vi "test_numpy.vi"() -> ()   [LabVIEW 2019]
uses:
  <vilib>/Analysis/Matrix/Datatypes/RealMatrix.ctl
  Ctrl/cmd_common.ctl
  <vilib>/Analysis/Matrix/Numeric/Add/Add (Elementwise) - RM,R.vi
  <vilib>/Analysis/Matrix/NI_Matrix.lvlib
  <vilib>/ptbypt/NI_PtbyPt.lvlib
panel:
  in  "sample length":i32=100
  out "Waveform Chart":cluster{dbl, dbl, "mean":dbl}(graph)
  in  "dt":u32
  in  "stop":bool
  in  "amplitude":dbl=1.0 format="%0.3f"
  out "first subarray":i32[](array[numeric])
  in  "Numeric":i32
  out "Real Matrix Element":dbl
  out "전치 행렬":T1
  out "열의 개수":i32
  out "크기 조정된 행렬":T1
  out "pw":T1=[[0.01, 0.01, 0.01, 0.01, 0.01, 0.01, 0.01, 0.01, 0.01, 0.01, 0.01, 0.01, 0.01, 0.01, 0.01, 0.01, 0.01, 0.01, 0.01, 0.01, 0.01, 0.01, 0.01, 0.01, 0.01, 0.01, 0.01, 0.01, 0.01, 0.01, 0.01, 0.01, 0.01, 0.01, 0.01, 0.01, 0.01, 0.01, 0.01, 0.01, 0.01, 0.01, 0.01, 0.01, 0.01, 0.01, 0.01, 0.01, 0.01, 0.01, 0.01, 0.01, 0.01, 0.01, 0.01, 0.01, 0.01, 0.01, 0.01, 0.01, 0.01, 0.01, 0.01, 0.01, 0.01, 0.01, 0.01, 0.01, 0.01, 0.01, 0.01, 0.01, 0.01, 0.01, 0.01, 0.01, 0.01, 0.01, 0.01, 0.01, 0.01, 0.01, 0.01, 0.01, 0.01, 0.01, 0.01, 0.01, 0.01, 0.01, 0.01, 0.01, 0.01, 0.01, 0.01, 0.01, 0.01, 0.01, 0.01, 0.01]]
  out "px":T1
  in  "NP":u32=100
  out "y 제곱근(x)":dbl
  out "x^y":dbl
  in  "**":dbl
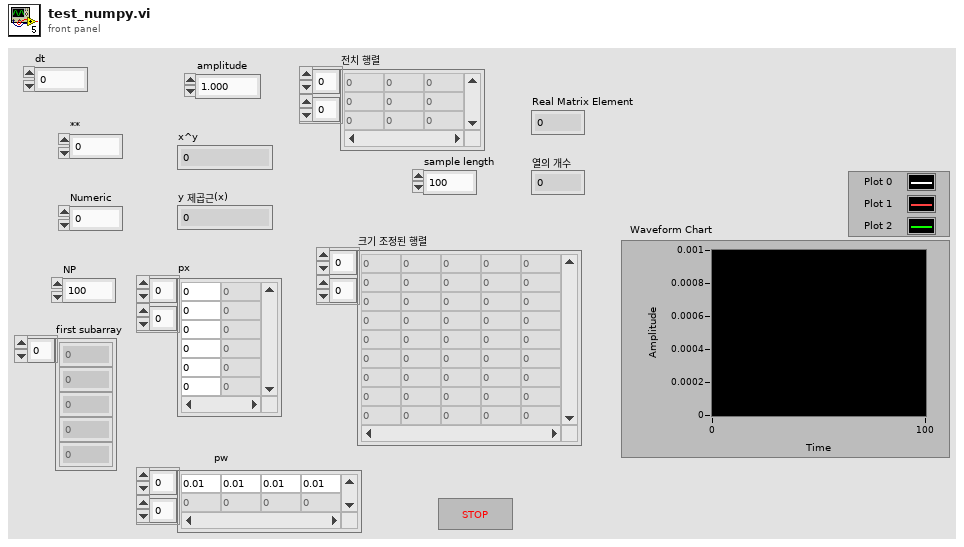
[diagram p1: front panel]
types:
  T1 = typedef "NI_Matrix.lvlib/RealMatrix.ctl" = dbl[][]
  T2 = typedef "cmd_common.ctl" = enum16{"read", "write"}
  T3 = cluster{"px":T1, "pw":T1, "x_dr":T1, "x_est":T1, "x_true":T1, "u":T1, "z":T1}
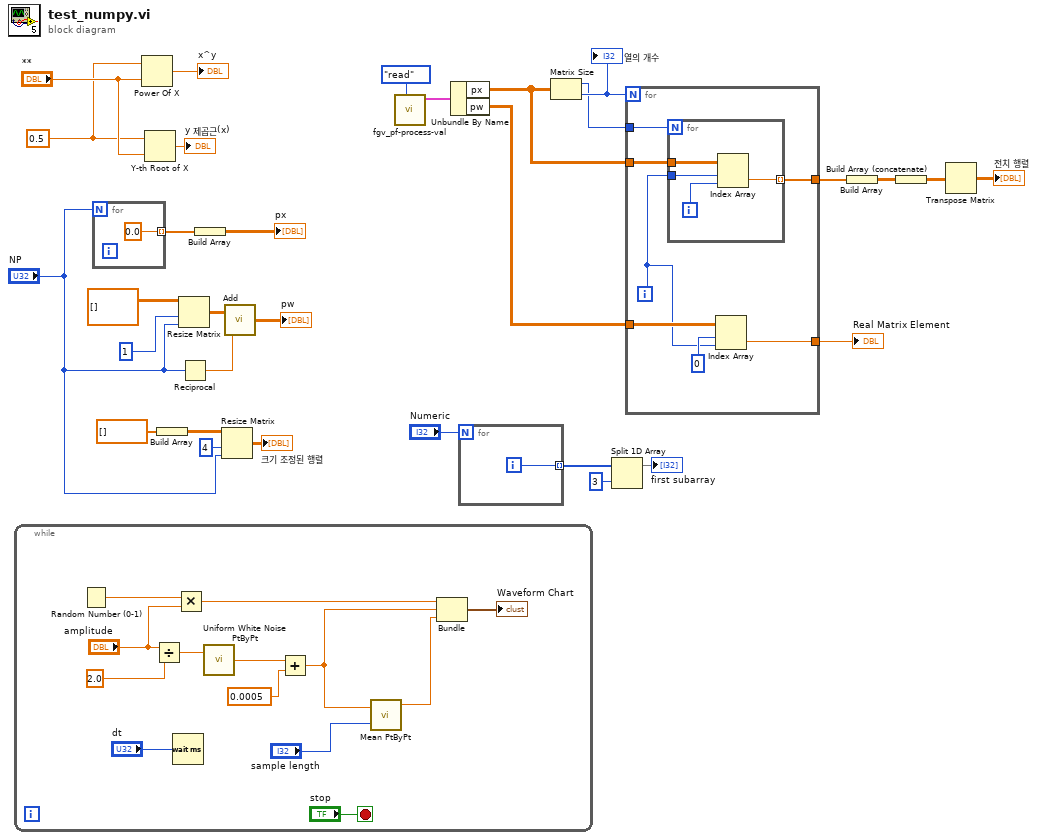
[diagram p0: block diagram]
diagram:
  w28 = 0.5 ("x")
  n1 = while {
    stop <- "stop" stop-if-true
    n2 = Random Number (0-1)() -> (number: 0 to 1=w44:dbl)
    n3 = Divide(x="amplitude", y=2.0) -> (x/y=w36:dbl)
    n4 = Wait (ms)(milliseconds to wait="dt") -> ()  [unwired: 1 out]
    n5 = Multiply(x=w44, y="amplitude") -> (x*y=w43:dbl)
    n6 = call <vilib>:"Uniform White Noise PtByPt.vi"("amplitude"=w36) -> ("uniform white noise"=w35:dbl)  [unwired: 2 in]
    n7 = Add(x=w35, y=0.0005) -> (x+y=w34:dbl)
    n8 = call <vilib>:"Mean PtByPt.vi"("x"=w34, "sample length"="sample length") -> ("mean"=w33:dbl)  [unwired: 2 in, 1 out]
    n9 = Bundle(w43, w34, "mean"=w33) -> (→"Waveform Chart":cluster{dbl, dbl, "mean":dbl})  [unwired: 1 in]
  }
  n10 = for {
    N: "NP" -> [_]
    tunnel: [0.0] -> w24 mode=indexing
  }
  n11 = Power Of X(1:"**", 2:w28) -> (0:→"x^y":dbl)
  n12 = Y-th Root of X(1:"**", 2:w28) -> (0:→"y 제곱근(x)":dbl)
  n13 = Build Array(dbl[] [] ("원소")) -> (w19:T1)
  n14 = Resize Matrix(1:"NP", 2:1 ("행의 개수"), 4:T1 [] ("행렬")) -> (0:w27:T1)
  n15 = Reciprocal(x="NP") -> (1/x=w26:dbl)
  n16 = Build Array(w24) -> (→"px":T1)
  n17 = Resize Matrix(1:"NP", 2:4 ("행의 개수"), 4:w19) -> (0:→"크기 조정된 행렬":T1)
  n18 = call-poly <vilib>:"Add.vi"("Real Scalar c"=w26, "Real Matrix A"=w27) -> ("A + c"=→"pw":T1)
  n19 = call "fgv_pf-process-val.vi"("cmd"=cmd_common."read") -> ("p-val out"=w13:T3)  [unwired: 10 in]
  n20 = Unbundle By Name(w13) -> ("px"=w12:T1, "pw"=w6:T1)
  n21 = for {
    N: "Numeric" -> [_]
    tunnel: [w46] -> w3 mode=indexing
    i -> [w46]
  }
  n22 = Matrix Size(0:w12) -> (1:w11:i32, 2:w15:i32)
  "열의 개수" <- w15
  n23 = Split 1D Array(array=w3, index=3) -> (first subarray=→"first subarray":i32[])  [unwired: 1 out]
  n24 = for {
    N: w15 -> [_]
    tunnel: w12 -> [w53]
    tunnel: w11 -> [w52]
    tunnel: [w51] -> w10
    tunnel: w6 -> [w49]
    tunnel: [w47] -> w5
    i -> [w48]
    n25 = for {
      N: w52 -> [_]
      tunnel: w53 -> [w57]
      tunnel: w48 -> [w55]
      tunnel: [w54] -> w51 mode=indexing
      i -> [w56]
      n26 = Index Array(array=w57, index (row)=w55, index (col)=w56) -> (element=w54:dbl)
    }
    n27 = Index Array(array=w49, index (row)=0 ("인덱스 (행)"), index (col)=w48) -> (element=w47:dbl)
  }
  "Real Matrix Element" <- w5
  n28 = Build Array(w10) -> (w7:dbl[][])
  n29 = Build Array (concatenate)(w7) -> (w9:T1)
  n30 = Transpose Matrix(1:w9) -> (0:→"전치 행렬":T1)
